vi "Initialize From Settings.vi"(8 "error in (no error)":errorcluster, 10 "settings":cluster{"key":string, "value":string}[](array[cluster]), 11 "Thread Configuration in":refnum<class "Thread Configuration.lvclass">) -> (0 "error out":errorcluster, 3 "Thread Configuration out":refnum<class "Thread Configuration.lvclass">)   [LabVIEW 2017, in "PXImc.lvlib" / "Thread Configuration.lvclass"]
uses:
  Thread Configuration.lvclass
  Thread Configuration.lvclass/Thread Configuration.ctl
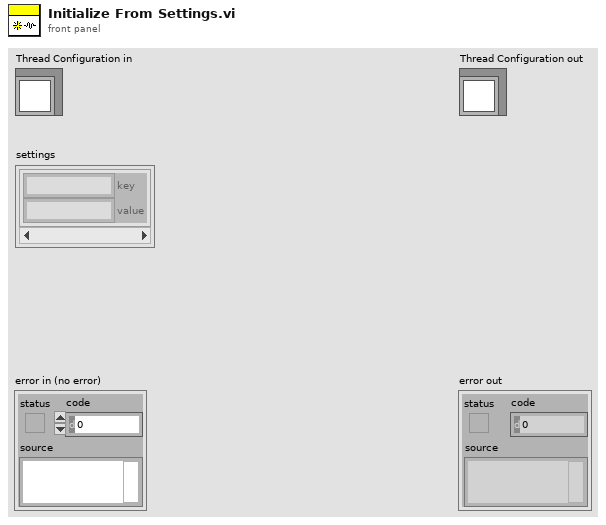
[diagram p1: front panel]
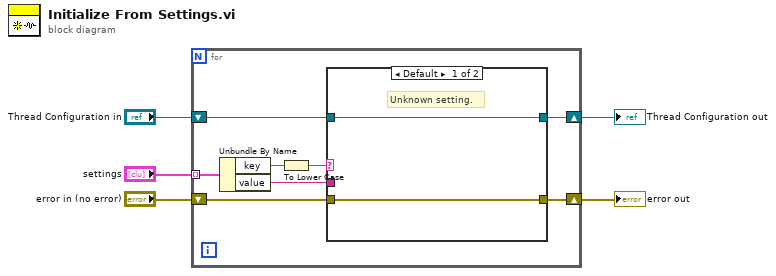
[diagram p0: block diagram]
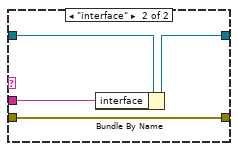
[diagram p2: hidden frame]
diagram:
  n1 = for {
    shift-right: [w9] -> w4
    shift-left: "error in (no error)" -> [w12]
    tunnel: "settings" -> [w13] mode=indexing
    shift-right: [w6] -> w1
    shift-left: "Thread Configuration in" -> [w7]
    n2 = Unbundle By Name(w13) -> ("key"=w11:string, "value"=w10:string)
    n3 = To Lower Case(string=w11) -> (all lower case string=w8:string)
    n4 = case shown="Default" w8 {
      tunnel: w12 -> [w15 w18]
      tunnel: w10 -> [_ w17]
      tunnel: [w15 w18] -> w9
      tunnel: w7 -> [w14 w19]
      tunnel: [w14 w16] -> w6
      frame Default {
        # "Unknown setting."
      }
      frame "interface" {
        n5 = Bundle By Name(cluster=w19, "interface"=w17) -> (w16:refnum<class "Thread Configuration.lvclass">)
      }
    }
  }
  "error out" <- w4
  "Thread Configuration out" <- w1
